vi "oa_Trigger r0 with Trigger Period.vi"(1 "trigger period [rev]":dbl=1.0, 2 "r0":dbl=1.0) -> (0 "triggered r0":dbl=1.0)   [LabVIEW 2017, in "SoundVib_OAUtility.lvlib"]
uses:
  <vilib>/addons/Sound and Vibration/Order Analysis/Utility/SoundVib_OAUtility.lvlib
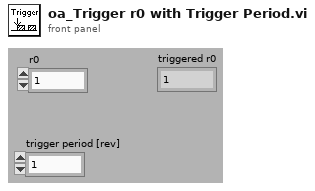
[diagram p1: front panel]
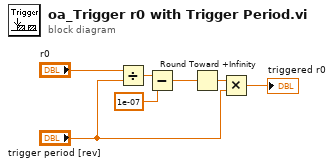
[diagram p0: block diagram]
diagram:
  n1 = Divide(x="r0", y="trigger period [rev]") -> (x/y=w5:dbl)
  n2 = Subtract(x=w5, y=1e-07) -> (x-y=w6:dbl)
  n3 = Round Toward +Infinity(x=w6) -> (ceil(x): smallest int >= x=w7:dbl)
  n4 = Multiply(x=w7, y="trigger period [rev]") -> (x*y=→"triggered r0":dbl)
